vi "Detect_Particle(Array)-2.vi"(0 "[IN] Sample Image":T2, 1 "[IN] AVI Refnum":T5, 2 "[IN] Particle Searching Settings":T4 {"Type of particle filter"."Measurement Parameter" items=["Center of Mass X", "Center of Mass Y", "First Pixel X", "First Pixel Y", "Bounding Rect Left", "Bounding Rect Top", "Bounding Rect Right", "Bounding Rect Bottom", "Max Feret Diameter Start X", "Max Feret Diameter Start Y", "Max Feret Diameter End X", "Max Feret Diameter End Y", "Max Horiz. Segment Length Left", "Max Horiz. Segment Length Right", "Max Horiz. Segment Length Row", "-", "Bounding Rect Width", "Bounding Rect Height", "Bounding Rect Diagonal", "Perimeter", "Convex Hull Perimeter", "Holes' Perimeter", "Max Feret Diameter", "Equivalent Ellipse Major Axis", "Equivalent Ellipse Minor Axis", "Equivalent Ellipse Minor Axis (Feret)", "Equivalent Rect Long Side", "Equivalent Rect Short Side", "Equivalent Rect Diagonal", "Equivalent Rect Short Side (Feret)", "Average Horiz. Segment Length", "Average Vert. Segment Length", "Hydraulic Radius", "Waddel Disk Diameter", "-", "Area", "Holes' Area", "Particle & Holes' Area", "Convex Hull Area", "Image Area", "-", "Number of Holes", "Number of Horiz. Segments", "Number of Vert. Segments", "-", "Orientation", "Max Feret Diameter Orientation", "-", "% Area/Image Area", "% Area/(Particle & Holes' Area)", "Ratio of Equivalent Ellipse Axes", "Ratio of Equivalent Rect Sides", "-", "Elongation Factor", "Compactness Factor", "Heywood Circularity Factor", "Type Factor", "-", "Sum X", "Sum Y", "Sum XX", "Sum XY", "Sum YY", "Sum XXX", "Sum XXY", "Sum XYY", "Sum YYY", "-", "Moment of Inertia XX", "Moment of Inertia XY", "Moment of Inertia YY", "Moment of Inertia XXX", "Moment of Inertia XXY", "Moment of Inertia XYY", "Moment of Inertia YYY", "Norm. Moment of Inertia XX", "Norm. Moment of Inertia XY", "Norm. Moment of Inertia YY", "Norm. Moment of Inertia XXX", "Norm. Moment of Inertia XXY", "Norm. Moment of Inertia XYY", "Norm. Moment of Inertia YYY", "Hu Moment 1", "Hu Moment 2", "Hu Moment 3", "Hu Moment 4", "Hu Moment 5", "Hu Moment 6", "Hu Moment 7"]}, 3 "Keep Nega-\ntive Values?":bool, 5 "[IN] Frame Number":u32, 7 "[IN] Destination Image":T2, 9 "[IN] Binarization Settings":cluster{"MinBin2":sgl, "MaxBin2":sgl}[](array[cluster]), 11 "error IN":errorcluster, 12 "[IN] # Channel":u8, 13 "[IN] Filtering Settings":T1) -> (6 "[OUT] Particle Reports (Pixels)":T6(array[cluster]) {"Orientation" format="%.2f"; "Dimensions"."Height" format="%.2f"; "Dimensions"."Width" format="%.2f"; "Center of Mass"."Y" format="%.2f"; "Center of Mass"."X" format="%.2f"; "Bounding Rect"."Bottom" format="%.2f"; "Bounding Rect"."Right" format="%.2f"; "Bounding Rect"."Top" format="%.2f"; "Bounding Rect"."Left" format="%.2f"; "Number of Holes" format="%.2f"; "Area" format="%.2f"}, 15 "error OUT":errorcluster)   [LabVIEW 2013]
uses:
  <vilib>/vision/Avi.llb/IMAQ AVI2 Refnum.ctl
  <vilib>/vision/Image Controls.llb/IMAQ Image.ctl
  <vilib>/vision/NI_Vision_Development_Module.lvlib
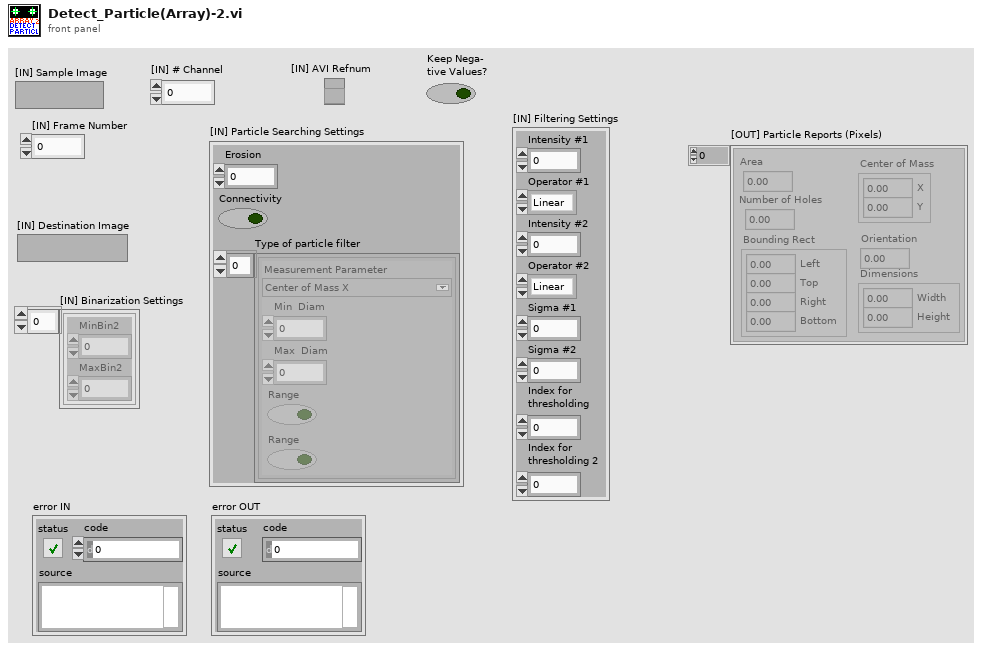
[diagram p1: front panel]
types:
  T1 = cluster{"Intensity #1":sgl, "Operator #1":enum32{"Linear", "Log", "Exp", "Square", "Square root", "Power X", "Power 1/X"}, "Intensity #2":sgl, "Operator #2":enum32{"Linear", "Log", "Exp", "Square", "Square root", "Power X", "Power 1/X"}, "Sigma #1":dbl, "Sigma #2":dbl, "Index for \nthresholding":u8, "Index for \nthresholding 2":u8}
  T2 = typedef "IMAQ Image.ctl" = refnum<image>
  T3 = typedef "Particle Parameters" = i32
  T4 = cluster{"Erosion":i32, "Connectivity ":bool, "Type of particle filter":cluster{"Measurement Parameter":T3, "Min  Diam":dbl, "Max  Diam":dbl, "Range":bool, "Range":bool}[]}
  T5 = typedef "IMAQ AVI2 Refnum.ctl" = refnum<k20>
  T6 = cluster{"Area":dbl, "Number of Holes":dbl, "Bounding Rect":cluster{"Left":dbl, "Top":dbl, "Right":dbl, "Bottom":dbl}, "Center of Mass":cluster{"X":dbl, "Y":dbl}, "Orientation":dbl, "Dimensions":cluster{"Width":dbl, "Height":dbl}}[]
  T7 = enum32{"Linear", "Log", "Exp", "Square", "Square root", "Power X", "Power 1/X"}
  T8 = cluster{"Starting Value":sgl, "Incremental Value":sgl, "Histogram":u32[]}
  T9 = cluster{"Measurement Parameter":T3, "Min  Diam":dbl, "Max  Diam":dbl, "Range":bool, "Range":bool}[]
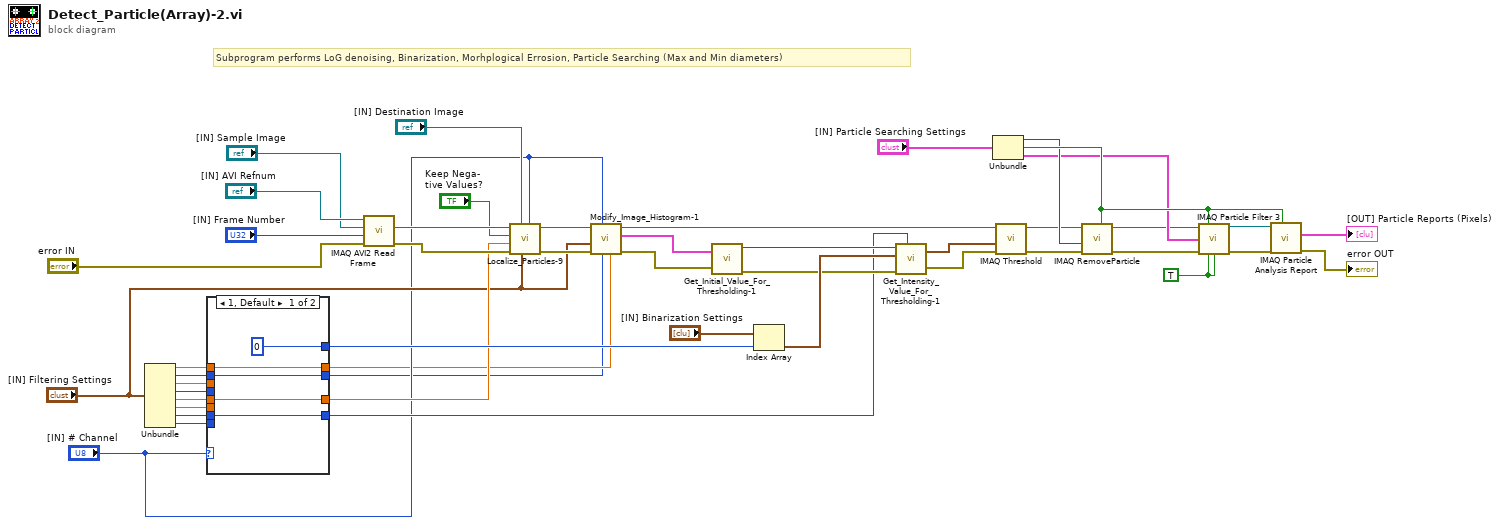
[diagram p0: block diagram]
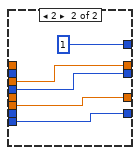
[diagram p2: hidden frame]
diagram:
  w47 = TRUE ("Fill Holes? (F)")
  # "Subprogram performs LoG denoising, Binarization, Morhplogical Errosion, Particle Searching (Max and Min diameters)"
  n1 = Unbundle("[IN] Filtering Settings") -> ("Intensity #1"=w9:sgl, "Operator #1"=w8:T7, "Intensity #2"=w7:sgl, "Operator #2"=w6:T7, "Sigma #1"=w21:dbl, "Sigma #2"=w22:dbl, "Index for \nthresholding"=w23:u8, "Index for \nthresholding 2"=w20:u8)
  n2 = case shown="1, Default" "[IN] # Channel" {
    tunnel: [0 1] -> w36
    tunnel: w23 -> [w50 _]
    tunnel: w22 -> [_ w56]
    tunnel: w21 -> [w51 _]
    tunnel: w20 -> [_ w55]
    tunnel: [w51 w56] -> w15
    tunnel: [w50 w55] -> w19
    tunnel: w9 -> [w49 _]
    tunnel: w8 -> [w48 _]
    tunnel: w7 -> [_ w54]
    tunnel: w6 -> [_ w53]
    tunnel: [w49 w54] -> w5
    tunnel: [w48 w53] -> w4
    frame 1, Default {
    }
    frame 2 {
    }
  }
  n3 = call "IMAQ AVI2 Read Frame"("error in (no error)"="error IN", "Frame Number"="[IN] Frame Number", "Image"="[IN] Sample Image", "AVI Refnum"="[IN] AVI Refnum") -> ("error out"=w17:errorcluster, "Image Out"=w18:T2)  [unwired: 5 in, 1 out]
  n4 = call "Localize_Particles-9.vi"("# channel"="[IN] # Channel", "[IN] Filtering Settings"="[IN] Filtering Settings", "[IN] Destination Image"="[IN] Destination Image", "error IN"=w17, "[IN] Sigma"=w15, "Keep Nega-\ntive Values?"="Keep Nega-\ntive Values?", "[IN] Frame"=w18) -> ("error OUT"=w12:errorcluster, "[OUT] LoG Processed Image"=w13:T2)  [unwired: 1 in, 1 out]
  n5 = call "Modify_Image_Histogram-1.vi"("[IN] Parameter"=w5, "[IN] Operator"=w4, "# channel"="[IN] # Channel", "error IN"=w12, "[IN] Filtering Settings"="[IN] Filtering Settings", "[IN] LoG Processed Image"=w13) -> ("error OUT"=w2:errorcluster, "[OUT] Histogram"=w3:T8, "[OUT] Histogram Modified Image"=w1:T2)  [unwired: 2 in, 1 out]
  n6 = call "Get_Initial_Value_For_Thresholding-1.vi"("[IN] Histogram Graph"=w3, "error IN"=w2) -> ("[OUT] Index of starting \npoint for thresholding"=w35:i32, "error OUT"=w33:errorcluster)  [unwired: 2 out]
  n7 = Index Array(array="[IN] Binarization Settings", index=w36) -> (element=w34:cluster{"MinBin2":sgl, "MaxBin2":sgl})
  n8 = call "Get_Intensity_Value_For_Thresholding-1.vi"("[IN] Index of starting \npoint for thresholding"=w35, "[IN] Thresholding range"=w34, "error IN"=w33, "[IN] Index for \nthresholding"=w19) -> ("[OUT] Thresholding range"=w32:cluster{"Lower value":sgl, "Upper value":sgl}, "error OUT"=w31:errorcluster)  [unwired: 1 in]
  n9 = Unbundle("[IN] Particle Searching Settings") -> ("Erosion"=w41:i32, "Connectivity"=w42:bool, "Type of particle filter"=w40:T9)
  n10 = call "IMAQ Threshold"("error in (no error)"=w31, "Range"=w32, "Image Src"=w1) -> ("error out"=w30:errorcluster, "Image Dst Out"=w29:T2)  [unwired: 7 in]
  n11 = call "IMAQ RemoveParticle"("Connectivity 4/8 (8)"=w42, "error in (no error)"=w30, "Number of Erosion"=w41, "Image Src"=w29) -> ("error out"=w38:errorcluster, "Image Dst Out"=w39:T2)  [unwired: 6 in]
  n12 = call "IMAQ Particle Filter 3"("Image Src"=w39, "Connectivity 4/8 (8)"=w42, "Selection Values"=w40, "error in (no error)"=w38, "Reject Border? (F)"=w47, "Fill Holes? (F)"=w47) -> ("Image Dst Out"=w46:T2, "error out"=w45:errorcluster)  [unwired: 7 in, 1 out]
  n13 = call "IMAQ Particle Analysis Report"("Connectivity 4/8 (8)"=w42, "error in (no error)"=w45, "Image"=w46) -> ("error out"=→"error OUT":errorcluster, "Particle Reports (Pixels)"=→"[OUT] Particle Reports (Pixels)":T6)  [unwired: 3 in, 4 out]
